vi "Build Timestamp.vi"(10 "timestamp low bits":u32, 11 "timestamp high bits":u32) -> (3 "timestamp out":dbl)   [LabVIEW 2020, in "AIM MIL-STD-1553 Engine.lvlib" / "Implementation.lvlib" / "Rx Execution Unit.lvclass"]
uses:
  Rx Execution Unit.lvclass
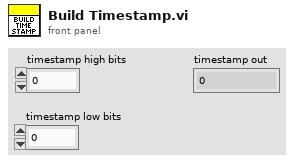
[diagram p1: front panel]
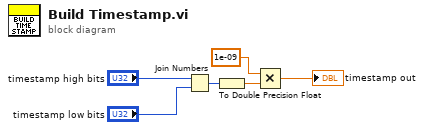
[diagram p0: block diagram]
diagram:
  n1 = Join Numbers(hi="timestamp high bits", lo="timestamp low bits") -> ((hi.lo)=w6:u64)
  n2 = To Double Precision Float(number=w6) -> (double precision float=w4:dbl)
  n3 = Multiply(x=1e-09 ("y"), y=w4) -> (x*y=→"timestamp out":dbl)
